vi "DGHD5331_virtualData.vi"() -> ()   [LabVIEW 2014]
uses:
  <vilib>/Utility/file.llb/Write To Spreadsheet File (string).vi
  <vilib>/Utility/file.llb/Write To Spreadsheet File (DBL).vi
panel:
  out "x*y":dbl
  out "Waveform Chart":cluster{i32, i32, i32, i32}(graph)
  out "concatenated string":string
  in  "Loop Timer":u32=500 min=500 max=5000 step=500
  in  "stop":bool
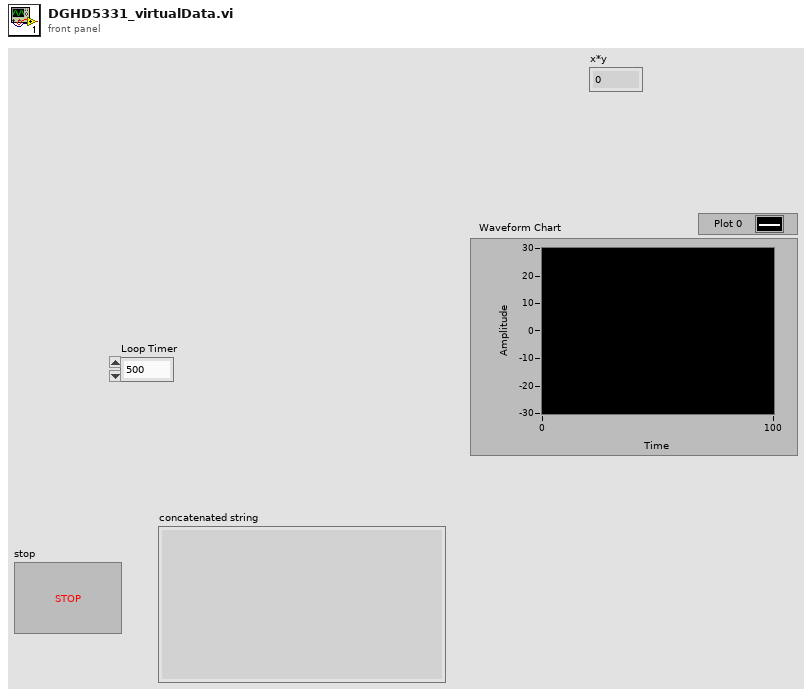
[diagram p1: front panel]
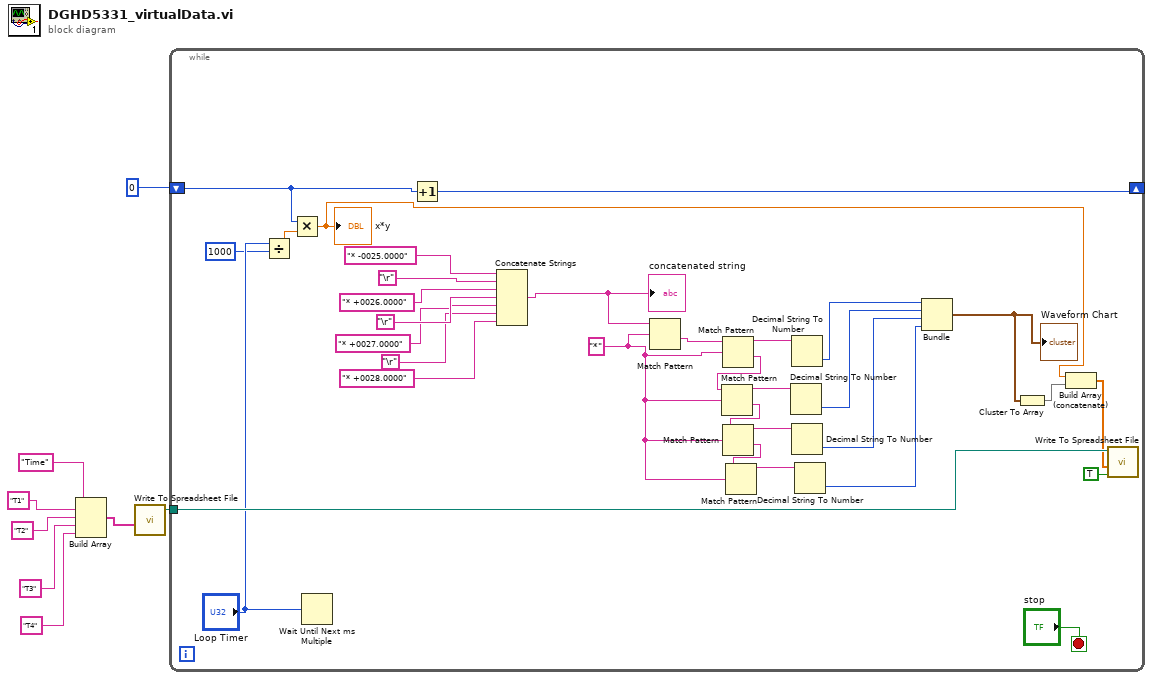
[diagram p0: block diagram]
diagram:
  n1 = Build Array("Time", "T1", "T2", "T3", "T4") -> (w4:string[])
  n2 = call-poly <vilib>:"Write To Spreadsheet File.vi"("1D data"=w4) -> ("new file path (Not A Path if cancelled)"=w3:path)  [unwired: 7 in]
  n3 = while {
    tunnel: w3 -> [w18]
    shift-right: [w15] -> _
    shift-left: 0 -> [w16]
    stop <- "stop" stop-if-true
    w24 = "*"
    n4 = Divide(x="Loop Timer", y=1000) -> (x/y=w12:dbl)
    n5 = Multiply(x=w16, y=w12) -> (x*y=w10:dbl)
    "x*y" <- w10
    n6 = Wait Until Next ms Multiple(millisecond multiple="Loop Timer") -> ()  [unwired: 1 out]
    n7 = Increment(x=w16) -> (x+1=w15:i32)
    n8 = Concatenate Strings("* -0025.0000", "\r", "* +0026.0000", "\r", "* +0027.0000", "\r", "* +0028.0000") -> (w33:string)
    "concatenated string" <- w33
    n9 = Match Pattern(string=w33, regular expression=w24) -> (after substring=w32:string)  [unwired: 1 in, 3 out]
    n10 = Match Pattern(string=w32, regular expression=w24) -> (before substring=w31:string, after substring=w29:string)  [unwired: 1 in, 2 out]
    n11 = Match Pattern(string=w29, regular expression=w24) -> (before substring=w30:string, after substring=w23:string)  [unwired: 1 in, 2 out]
    n12 = Match Pattern(string=w23, regular expression=w24) -> (before substring=w26:string, after substring=w22:string)  [unwired: 1 in, 2 out]
    n13 = Match Pattern(string=w22, regular expression=w24) -> (before substring=w25:string)  [unwired: 1 in, 3 out]
    n14 = Decimal String To Number(string=w30) -> (number=w27:i32)  [unwired: 2 in, 1 out]
    n15 = Decimal String To Number(string=w31) -> (number=w28:i32)  [unwired: 2 in, 1 out]
    n16 = Decimal String To Number(string=w26) -> (number=w21:i32)  [unwired: 2 in, 1 out]
    n17 = Decimal String To Number(string=w25) -> (number=w20:i32)  [unwired: 2 in, 1 out]
    n18 = Bundle(w28, w27, w21, w20) -> (w19:cluster{i32, i32, i32, i32})  [unwired: 1 in]
    "Waveform Chart" <- w19
    n19 = Cluster To Array(cluster=w19) -> (array=w11:i32[])
    n20 = Build Array (concatenate)(w10, w11) -> (w9:dbl[])
    n21 = call-poly <vilib>:"Write To Spreadsheet File.vi"("append to file? (new file:F)"=TRUE, "1D data"=w9, "file path (dialog if empty)"=w18) -> ()  [unwired: 5 in, 1 out]
  }
